vi "Get last row.vi"(1 "Data input file":path) -> (0 "last row":string[](array[string]))   [LabVIEW 2015]
uses:
  <vilib>/Utility/file.llb/Read From Spreadsheet File (string).vi
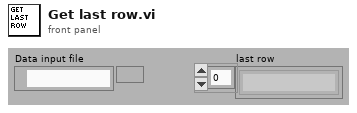
[diagram p1: front panel]
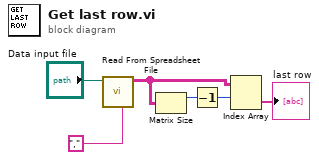
[diagram p0: block diagram]
diagram:
  n1 = call-poly <vilib>:"Read From Spreadsheet File.vi"("delimiter (\\t)"="," ("delimiter (\\t)"), "file path (dialog if empty)"="Data input file") -> ("all rows"=w5:string[][])  [unwired: 5 in, 4 out]
  n2 = Matrix Size(0:w5) -> (1:w2:i32)  [unwired: 1 out]
  n3 = Decrement(x=w2) -> (x-1=w1:i32)
  n4 = Index Array(array=w5, index (row)=w1) -> (element=→"last row":string[])  [unwired: 1 in]
